vi "VisaWriteforPumps.vi"(8 "error in (no error)":errorcluster, 9 "Command:":string, 10 "Pump Address":enum16{"00", "01", "02", "03"}(ring), 11 "VISA Refnum in":refnum<visa-resource-name>) -> (0 "error out":errorcluster, 3 "VISA Refnum out":refnum<visa-resource-name>)   [LabVIEW 2014]
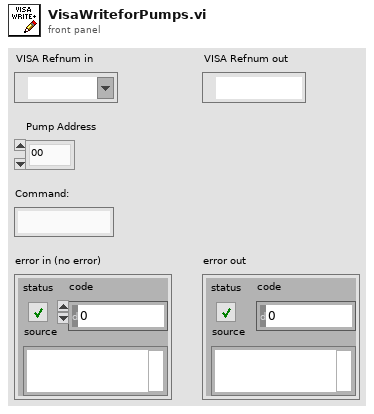
[diagram p1: front panel]
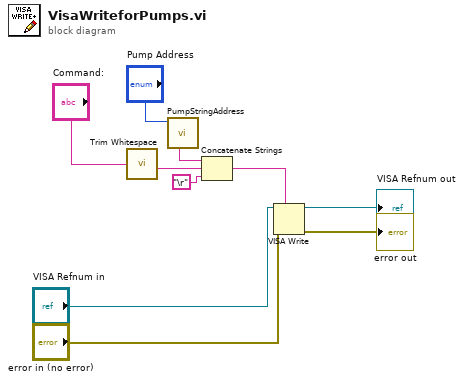
[diagram p0: block diagram]
diagram:
  n1 = call <vilib>:"Trim Whitespace.vi"("string"="Command:") -> ("trimmed string"=w3:string)  [unwired: 1 in]
  n2 = call "PumpStringAddress.vi"("Pump Address"="Pump Address") -> ("String"=w2:string)  [unwired: 10 in]
  n3 = Concatenate Strings(w2, w3, "\r") -> (w1:string)
  n4 = VISA Write(VISA resource name="VISA Refnum in", write buffer=w1, error in (no error)="error in (no error)") -> (VISA resource name out=→"VISA Refnum out":refnum<visa-resource-name>, error out=→"error out":errorcluster)  [unwired: 1 out]
